vi "I-O Test.vi"() -> ()   [LabVIEW 2016]
uses:
  Classes/Controller/I-O/I-O.lvclass
  Classes/Controller/Controller.lvclass
panel:
  in  "Tab Control":enum32{"assembly valve", "IO test"}(tab)
  out "channel":dbl
  out "Value 2":bool=TRUE
  in  "Type":i32
  in  "Position":i32
  in  "Region":i32
  in  "Value":bool=TRUE
  in  "values":bool[](array[boolean])
  in  "indices":i32[](array[numeric])
  out "Array 2":bool[](array[boolean])
  in  "Stop":bool
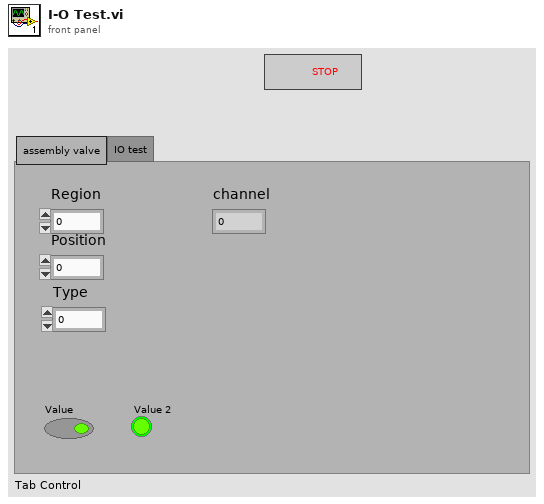
[diagram p1: front panel]
types:
  T1 = typedef "Controller.lvclass/Controllers.ctl" = cluster{"I-O.lvclass":refnum<class "I-O.lvclass">, "Motion.lvclass":refnum<class "Motion.lvclass">, "Dispenser.lvclass":refnum<class "Dispenser.lvclass">}
  T2 = typedef "I-O.lvclass/Pin Map.ctl" = cluster{"Region Valves":i32[], "Extra Valves":dbl[][][], "Tool Primary Valve":i32, "Tool Secondary Valve":i32, "Region Sensors":i32[], "Extra Sensors":dbl[][][], "Tool Primary Sensor":dbl, "Tool Secondary Sensor":dbl, "Compression Sensor":dbl, "5V":i32}
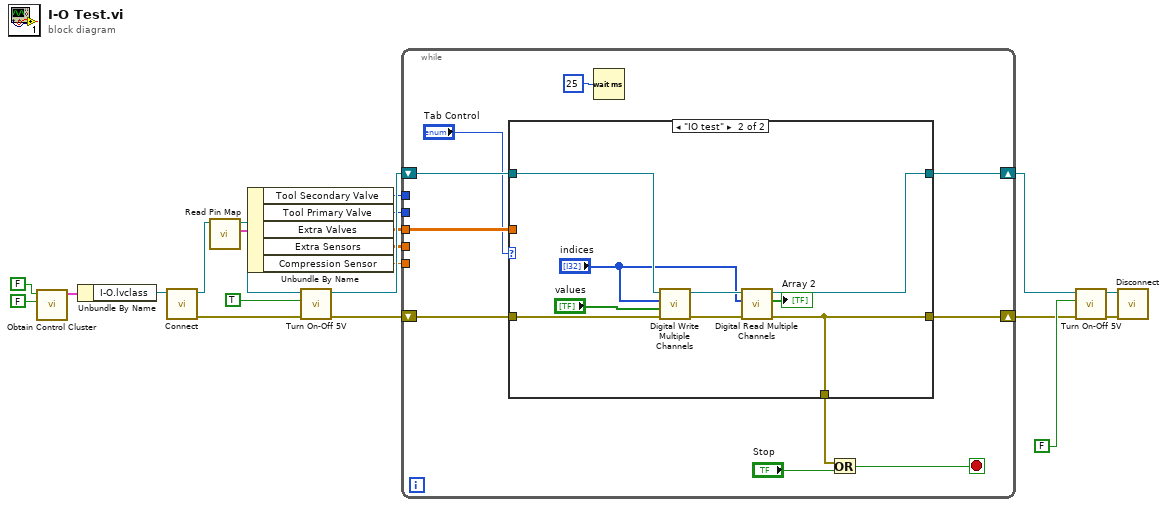
[diagram p0: block diagram]
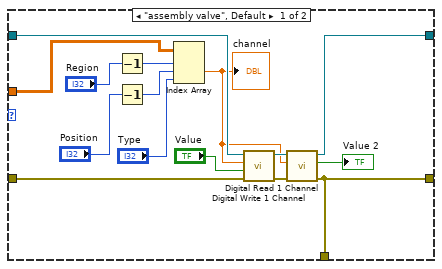
[diagram p2: hidden frame]
diagram:
  n1 = call "Obtain Control Cluster.vi"("Dispense"=FALSE, "Motion"=FALSE) -> ("Control Out"=w5:T1)  [unwired: 9 in]
  n2 = Unbundle By Name(w5) -> ("I-O.lvclass"=w4:refnum<class "I-O.lvclass">)
  n3 = call-dynamic "Connect.vi"("Controller in"=w4) -> ("error out"=w12:errorcluster, "Controller out"=w14:refnum<class "I-O.lvclass">)  [unwired: 9 in]
  n4 = call-dynamic "Read Pin Map.vi"("I-O in"=w14) -> ("Pin Map 2"=w16:T2, "I-O out"=w15:refnum<class "I-O.lvclass">)  [unwired: 8 in, 1 out]
  n5 = Unbundle By Name(w16) -> ("Tool Secondary Valve"=w2:i32, "Tool Primary Valve"=w1:i32, "Extra Valves"=w8:dbl[][][], "Extra Sensors"=w13:dbl[][][], "Compression Sensor"=w3:dbl)
  n6 = call-dynamic "Turn On-Off 5V.vi"("error in (no error)"=w12, "Value"=TRUE, "I-O in"=w15) -> ("error out"=w11:errorcluster, "I-O out"=w21:refnum<class "I-O.lvclass">)  [unwired: 7 in]
  n7 = while {
    shift-right: [w25] -> w18
    shift-left: w21 -> [w27]
    tunnel: w13 -> [_]
    shift-right: [w22] -> w10
    shift-left: w11 -> [w26]
    tunnel: w8 -> [w28]
    tunnel: w3 -> [_]
    tunnel: w2 -> [_]
    tunnel: w1 -> [_]
    stop <- w29 stop-if-true
    n8 = case shown="\"IO test\"" "Tab Control" {
      tunnel: w28 -> [w46 _]
      tunnel: w27 -> [w45 w55]
      tunnel: w26 -> [w44 w54]
      tunnel: [w37 w50] -> w25
      tunnel: [w32 w52] -> w24
      tunnel: [w32 w52] -> w22
      frame "assembly valve", Default {
        n9 = Decrement(x="Region") -> (x-1=w42:i32)
        n10 = Decrement(x="Position") -> (x-1=w39:i32)
        n11 = Index Array(array=w46, index (dim 0)=w42, index (dim 1)=w39, index (dim 2)="Type") -> (element=w35:dbl)
        "channel" <- w35
        n12 = call-dynamic "Digital Write 1 Channel.vi"("error constant"=w44, "Value"="Value", "Channel"=w35, "I-O.lvclass"=w45) -> ("error IO"=w33:errorcluster, "I-O.lvclass 2"=w36:refnum<class "I-O.lvclass">)  [unwired: 6 in]
        n13 = call-dynamic "Digital Read 1 Channel.vi"("error in (no error)"=w33, "Read"=w35, "I-O in"=w36) -> ("error out"=w32:errorcluster, "Value"=→"Value 2":bool, "I-O out"=w37:refnum<class "I-O.lvclass">)  [unwired: 6 in]
      }
      frame "IO test" {
        n14 = call-dynamic "Digital Write Multiple Channels.vi"("error in (no error)"=w54, "values"="values", "indices"="indices", "I-O in"=w55) -> ("error out"=w53:errorcluster, "I-O out"=w51:refnum<class "I-O.lvclass">)  [unwired: 6 in]
        n15 = call-dynamic "Digital Read Multiple Channels.vi"("error in (no error)"=w53, "indices"="indices", "I-O in"=w51) -> ("error out"=w52:errorcluster, "Array 2"=→"Array 2":bool[], "I-O out"=w50:refnum<class "I-O.lvclass">)  [unwired: 6 in]
      }
    }
    n16 = Wait (ms)(milliseconds to wait=u32 25) -> ()  [unwired: 1 out]
    n17 = Or(x=w24, y="Stop") -> (x .or. y?=w29:bool)
  }
  n18 = call-dynamic "Turn On-Off 5V.vi"("error in (no error)"=w10, "Value"=FALSE, "I-O in"=w18) -> ("error out"=w9:errorcluster, "I-O out"=w19:refnum<class "I-O.lvclass">)  [unwired: 7 in]
  n19 = call-dynamic "Disconnect.vi"("error in (no error)"=w9, "I-O in"=w19) -> ()  [unwired: 8 in, 1 out]
